vi "set_Power.vi"(8 "error in (no error)":errorcluster, 9 "Power":i32, 10 "LASER ON":bool, 11 "VISA resource name":refnum<visa-resource-name>) -> (0 "error out":errorcluster, 3 "VISA resource name out":refnum<visa-resource-name>)   [LabVIEW 2013]
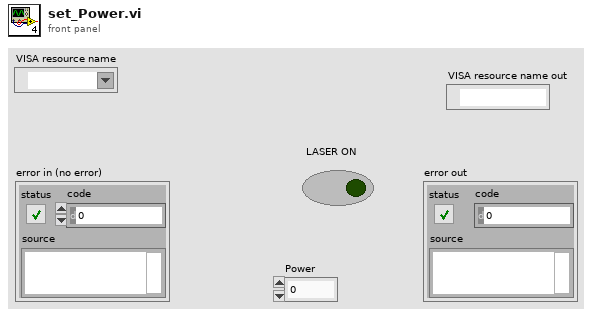
[diagram p1: front panel]
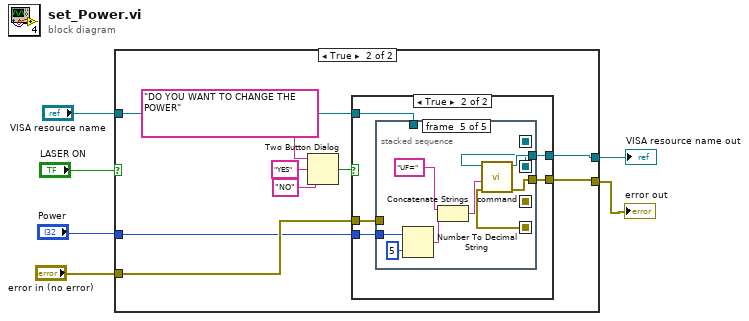
[diagram p0: block diagram]
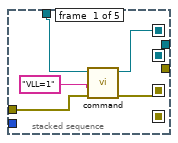
[diagram p4: hidden frame]
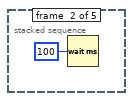
[diagram p5: hidden frame]
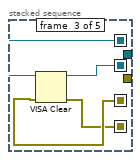
[diagram p6: hidden frame]
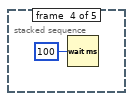
[diagram p7: hidden frame]
diagram:
  n1 = case shown="True" "LASER ON" {
    tunnel: "error in (no error)" -> [w7 w13]
    tunnel: "VISA resource name" -> [w8 w12]
    tunnel: [w8 w11] -> w3
    tunnel: [w7 w10] -> w2
    tunnel: "Power" -> [_ w9]
    frame False {
    }
    frame True {
      n2 = Two Button Dialog(message="DO YOU WANT TO CHANGE THE POWER", 1:"NO" ("F button name (\"Cancel\")"), 2:"YES" ("T button name (\"OK\")")) -> (T button?=w17:bool)
      n3 = case shown="True" w17 {
        tunnel: w13 -> [w18 w24]
        tunnel: w12 -> [w19 w23]
        tunnel: [w19 w22] -> w11
        tunnel: [w18 w21] -> w10
        tunnel: w9 -> [_ w20]
        frame False {
        }
        frame True {
          n4 = stacked-sequence {
            seq-local: [w27 _ _ _ _] -> [_ _ w33 _ _]
            seq-local: [w26 _ _ _ _] -> [_ _ w34 _ _]
            seq-local: [_ _ w32 _ _] -> [_ _ _ _ w37]
            seq-local: [_ _ w31 _ _] -> [_ _ _ _ w36]
            tunnel: w24 -> [w28 _ _ _ _]
            tunnel: w23 -> [w29 _ _ _ _]
            tunnel: [_ _ _ _ w44] -> w22
            tunnel: [_ _ _ _ w43] -> w21
            tunnel: w20 -> [_ _ _ _ w38]
            frame #0 {
              n5 = call "command.vi"("error in (no error)"=w28, "write buffer"="VLL=1", "VISA resource name"=w29) -> ("error out"=w27:errorcluster, "VISA resource name out"=w26:refnum<visa-resource-name>)  [unwired: 7 in]
            }
            frame #1 {
              n6 = Wait (ms)(milliseconds to wait=u32 100) -> ()  [unwired: 1 out]
            }
            frame #2 {
              n7 = VISA Clear(VISA resource name=w34, error in (no error)=w33) -> (VISA resource name out=w31:refnum<visa-resource-name>, error out=w32:errorcluster)
            }
            frame #3 {
              n8 = Wait (ms)(milliseconds to wait=u32 100) -> ()  [unwired: 1 out]
            }
            frame #4 {
              n9 = Number To Decimal String(number=w38, width (-)=i16 5) -> (decimal integer string=w41:string)
              n10 = Concatenate Strings("UF=" ("write buffer"), w41) -> (w40:string)
              n11 = call "command.vi"("error in (no error)"=w37, "write buffer"=w40, "VISA resource name"=w36) -> ("error out"=w43:errorcluster, "VISA resource name out"=w44:refnum<visa-resource-name>)  [unwired: 7 in]
            }
          }
        }
      }
    }
  }
  "VISA resource name out" <- w3
  "error out" <- w2
